vi "Save To File (PDM).vi"(8 "error in (no error)":errorcluster, 10 "PDM input settings":T1={"PDM clock rate"=51200.0, "decimation factor"=1, "bit clock direction"=enum."In", "logic level"=enum."3.3 V"} {"decimation factor" items=["24"=24, "32"=32, "48"=48, "64"=64, "96"=96, "128"=128]; "PDM clock rate" format="%#_6p"}, 11 "file path":path) -> (0 "error out":errorcluster)   [LabVIEW 2022 SP3, in "input cfg file.lvlib"]
uses:
  input cfg file.lvlib
  controls/PDM/PDM input settings.ctl
  <vilib>/PDM Acquisition Toolkit/shared/controls/decimation order.ctl
  controls/bit clock direction.ctl
  <vilib>/PDM Acquisition Toolkit/host/Classes/Session/Controls/Logic Levels.ctl
  controls/input type.ctl
  PDM/PDM input cfg file.lvlib
  <vilib>/PDM Acquisition Toolkit/host/Classes/Session/DecoderSession.lvclass
  <vilib>/PDM Acquisition Toolkit/shared/PDM Shared.lvlib
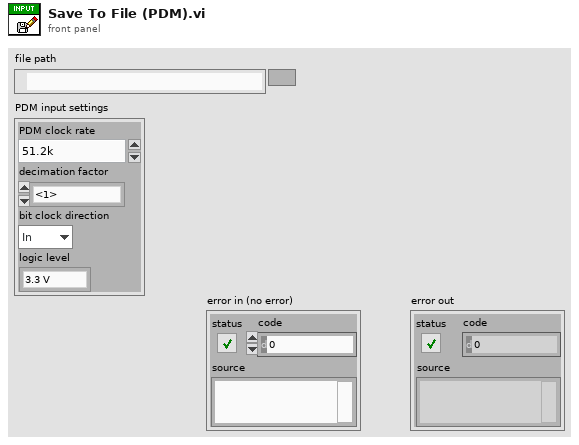
[diagram p1: front panel]
types:
  T1 = typedef "PDM input settings.ctl" = cluster{"PDM clock rate":dbl, "decimation factor":T2, "bit clock direction":T3, "logic level":T4}
  T2 = typedef "PDM Shared.lvlib/decimation order.ctl" = u16
  T3 = typedef "bit clock direction.ctl" = enum32{"In", "Out"}
  T4 = typedef "PDM Acquisition Class Library.lvlib/DecoderSession.lvclass/Logic Levels.ctl" = enum16{"3.3 V", "1.8 V", "1.2 V"}
  T5 = typedef "input type.ctl" = enum32{"Digital Serial", "PDM"}
  T6 = typedef "PDM input settings_json.ctl" = cluster{"PDM clock rate":dbl, "decimation factor":dbl, "bit clock direction":string, "logic level":string}
  T7 = enum16{"open", "replace", "create", "open or create", "replace or create", "replace or create with confirmation"}
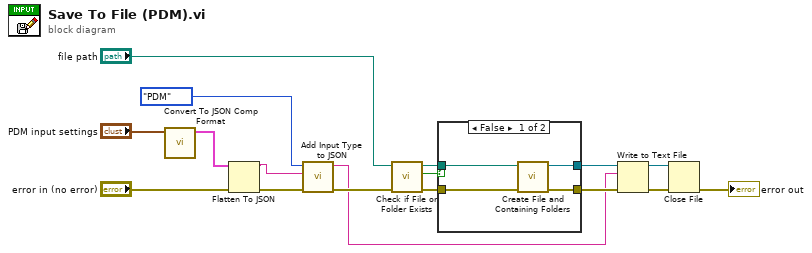
[diagram p0: block diagram]
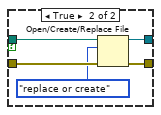
[diagram p2: hidden frame]
diagram:
  n1 = call "Convert To JSON Comp Format.vi"("input settings"="PDM input settings") -> ("input settings JSON"=w1:cluster{"PDM":T6})  [unwired: 10 in]
  n2 = Flatten To JSON(anything=w1, error in (no error)="error in (no error)") -> (JSON string=w5:string, 11:w7:errorcluster)  [unwired: 1 in]
  n3 = call "Add Input Type to JSON.vi"("error in (no error)"=w7, "input cfg JSON"=w5, "input type"=input_type."PDM") -> ("error out"=w6:errorcluster, "input cfg JSON"=w4:string)  [unwired: 7 in]
  n4 = call <vilib>:"Check if File or Folder Exists.vi"("error in (no error)"=w6, "path"="file path") -> ("error out"=w10:errorcluster, "file or folder exists?"=w9:bool, "dup path"=w8:path)  [unwired: 7 in]
  n5 = case shown="False" w9 {
    tunnel: [w21 w26] -> w16
    tunnel: [w20 w23] -> w15
    tunnel: w10 -> [w19 w24]
    tunnel: w8 -> [w18 w25]
    frame False {
      n6 = call <vilib>:"Create File and Containing Folders.vi"("error in (no error)"=w19, "file path"=w18) -> ("error out"=w21:errorcluster, "refnum out"=w20:refnum<file>)  [unwired: 8 in]
    }
    frame True {
      n7 = Open/Create/Replace File(file path (use dialog)=w25, error in=w24, operation (0:open)=T7."replace or create") -> (refnum out=w23:refnum<file>, error out=w26:errorcluster)  [unwired: 3 in, 1 out]
    }
  }
  n8 = Write to Text File(file (use dialog)=w15, text=w4, error in=w16) -> (refnum out=w13:refnum<file>, error out=w14:errorcluster)  [unwired: 1 in, 1 out]
  n9 = Close File(refnum=w13, error in=w14) -> (error out=→"error out":errorcluster)  [unwired: 1 out]
